vi "Power - Finite Measurement.vi"() -> ()   [LabVIEW 2022 SP3]
doc: "This example demonstrates how to acquire a single buffer of power measurements using a DAQmx device.\n\nFor instructions on how to connect your signals to the DAQ device, refer to your device documentation."
uses:
  <vilib>/Utility/error.llb/DialogType.ctl
  <vilib>/DAQmx/read.llb/DAQmx Read (Power 1D DBL 1Chan NSamp).vi
  <vilib>/DAQmx/create/channels.llb/DAQmx Create Channel (Power).vi
  <vilib>/DAQmx/configure/timing.llb/DAQmx Timing (Sample Clock).vi
  <vilib>/DAQmx/configure/trigger.llb/DAQmx Start Trigger (Digital Edge).vi
  <vilib>/DAQmx/configure/trigger.llb/DAQmx Reference Trigger (Digital Edge).vi
  <vilib>/DAQmx/miscellaneous.llb/DAQmx Fill In Error Info.vi
  <resource>/objmgr/daqmx.rc
panel:
  out "Current Waveform Graph":dbl[](graph)
  in  "Remote Sense":i32(ring)=16095 items=["Local"=16095, "Remote"=16096]
  in  "Idle Output Behavior":i32(ring)=15503 items=["Output Disabled"=15503, "Maintain Existing Value"=12528]
  in  "Output Enable":bool=TRUE
  in  "Trigger Type":T1(tab)
  in  "Digital Start Trigger Edge":i32(ring)=10280 caption="Edge" items=["Rising"=10280, "Falling"=10171]
  in  "Digital Start Trigger Source":tag="/TS1Mod2/PFI0" caption="Source"
  in  "Digital Pause Trigger Pause When":i32(ring)=10192 caption="Pause When" items=["High"=10192, "Low"=10214]
  in  "Digital Pause Trigger Source":tag="/TSMod2/PFI0" caption="Source"
  in  "Digital Reference Trigger Source":tag="/TSMod2/PFI0" caption="Source"
  in  "Digital Reference Trigger Edge":i32(ring)=10280 caption="Edge" items=["Rising"=10280, "Falling"=10171]
  in  "Digital Reference Pretrigger Samples":u32=500 caption="Pretrigger Samples"
  in  "Number of Samples":i32=100
  in  "Sample Rate":dbl=1000.0
  in  "Sample Clock Source":tag="OnboardClock"
  in  "Voltage Setpoint":dbl=6.0
  in  "Current Setpoint":dbl=3.0
  in  "Physical Channel":tag="TS1Mod1/power"
  out "Actual Sample Rate":dbl=1000.0 format="%0.2f"
  out "Voltage Waveform Graph":dbl[](graph)
  # "Channel Settings"
  # "Acquired Voltage Data"
  # "Acquired Current Data"
  # "Timing Settings"
  # "Trigger Settings"
  # "To enable triggers, select a tab above, and configure the settings.\n\nNot all hardware supports all trigger types. Refer to your device documentation for more information."
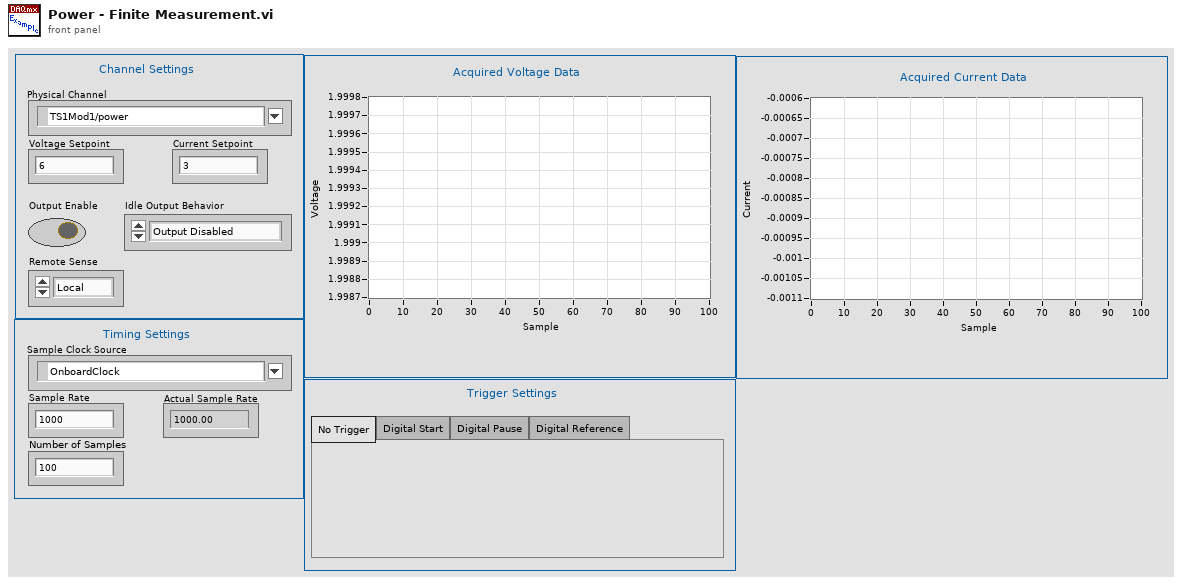
[diagram p1: front panel]
types:
  T1 = enum32{"No Trigger", "Digital Start", "Digital Pause", "Digital Reference"}
  T2 = typedef "DialogType.ctl" = u16
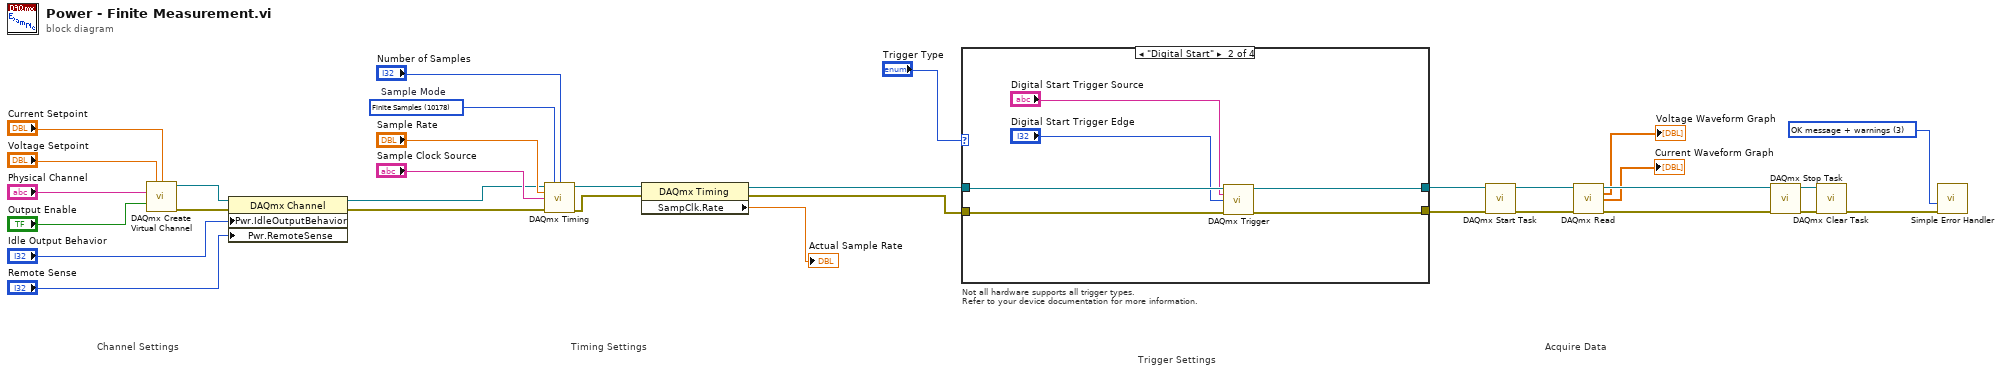
[diagram p0: block diagram]
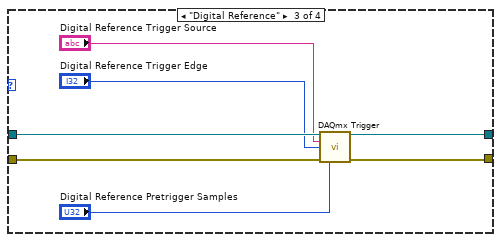
[diagram p3: hidden frame]
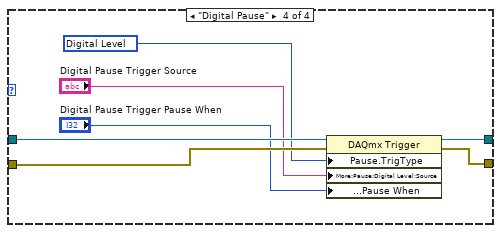
[diagram p4: hidden frame]
diagram:
  w13 = T2 3 items=["no dialog", "OK message", "continue or stop message", "OK message + warnings", "continue/stop + warnings"] ("type of dialog (OK msg:1)")
  w30 = 10178 items=["Finite Samples"=10178, "Continuous Samples"=10123, "Hardware Timed Single Point"=12522]  # Sample Mode
  # "Not all hardware supports all trigger types.\nRefer to your device documentation for more information."
  # "Trigger Settings"
  # "Acquire Data"
  # "Timing Settings"
  # "Channel Settings"
  n1 = call-poly <vilib>:"DAQmx Create Virtual Channel.vi"("voltage setpoint"="Voltage Setpoint", "current setpoint"="Current Setpoint", "physical channels"="Physical Channel", "output enable"="Output Enable") -> ("task out"=w6:refnum<k21>, "error out"=w7:errorcluster)  [unwired: 10 in]
  n2 = property class="DAQmx Channel"(reference=w6, error in=w7, "Pwr.IdleOutputBehavior"="Idle Output Behavior", "Pwr.RemoteSense"="Remote Sense") -> (reference out=w4:refnum<k21>, error out=w5:errorcluster)
  n3 = call-poly <vilib>:"DAQmx Timing.vi"("task/channels in"=w4, "sample mode"=w30, "samples per channel"="Number of Samples", "rate"="Sample Rate", "source"="Sample Clock Source", "error in"=w5) -> ("task out"=w32:refnum<k21>, "error out"=w31:errorcluster)  [unwired: 8 in]
  n4 = property class="DAQmx Timing"(reference=w32, error in=w31) -> (reference out=w29:refnum<k21>, error out=w28:errorcluster, "SampClk.Rate"=→"Actual Sample Rate":dbl)
  n5 = case shown="\"Digital Start\"" "Trigger Type" {
    tunnel: w29 -> [w34 w40 w47 w54]
    tunnel: w28 -> [w33 w39 w46 w51]
    tunnel: [w34 w38 w45 w53] -> w11
    tunnel: [w33 w37 w44 w52] -> w10
    frame "No Trigger", Default {
    }
    frame "Digital Start" {
      n6 = call-poly <vilib>:"DAQmx Trigger.vi"("task/channels in"=w40, "source"="Digital Start Trigger Source", "edge"="Digital Start Trigger Edge", "error in"=w39) -> ("task out"=w38:refnum<k21>, "error out"=w37:errorcluster)  [unwired: 10 in]
    }
    frame "Digital Reference" {
      n7 = call-poly <vilib>:"DAQmx Trigger.vi"("task/channels in"=w47, "source"="Digital Reference Trigger Source", "edge"="Digital Reference Trigger Edge", "error in"=w46, "pretrigger samples per channel"="Digital Reference Pretrigger Samples") -> ("task out"=w45:refnum<k21>, "error out"=w44:errorcluster)  [unwired: 9 in]
    }
    frame "Digital Pause" {
      w50 = 10152 items=["Analog Level"=10101, "Analog Window"=10103, "Digital Level"=10152, "Digital Pattern"=10398, "None"=10230] ("Pause.TrigType")
      n8 = property class="DAQmx Trigger"(reference=w54, error in=w51, "Pause.TrigType"=w50, "More:Pause:Digital Level:Source"="Digital Pause Trigger Source", "More:Pause:Digital Level:Pause When"="Digital Pause Trigger Pause When") -> (reference out=w53:refnum<k21>, error out=w52:errorcluster)
    }
  }
  n9 = call <vilib>:"DAQmx Start Task.vi"("task/channels in"=w11, "error in"=w10) -> ("task out"=w27:refnum<k21>, "error out"=w26:errorcluster)  [unwired: 12 in]
  n10 = call-poly <vilib>:"DAQmx Read.vi"("task/channels in"=w27, "error in"=w26) -> ("task out"=w15:refnum<k21>, "voltage"=→"Voltage Waveform Graph":dbl[], "current"=→"Current Waveform Graph":dbl[], "error out"=w14:errorcluster)  [unwired: 10 in]
  n11 = call <vilib>:"DAQmx Stop Task.vi"("task/channels in"=w15, "error in"=w14) -> ("task out"=w17:refnum<k21>, "error out"=w16:errorcluster)  [unwired: 12 in]
  n12 = call <vilib>:"DAQmx Clear Task.vi"("task in"=w17, "error in"=w16) -> ("error out"=w25:errorcluster)  [unwired: 13 in]
  n13 = call <vilib>:"Simple Error Handler.vi"("type of dialog (OK msg:1)"=w13, "error in (no error)"=w25) -> ()  [unwired: 3 in, 5 out]
